vi "exprand1Lars.vi"() -> ()   [LabVIEW 2010]
uses:
  <vilib>/Analysis/NI_AALBase.lvlib
panel:
  out "Waveform Graph of random numbers":dbl[](graph)
  in  "Histogram intervals":i32
  out "Histogram":T1(graph)
  in  "Desired Expected Random Number":dbl
  in  "Number of Random Numbers":i32
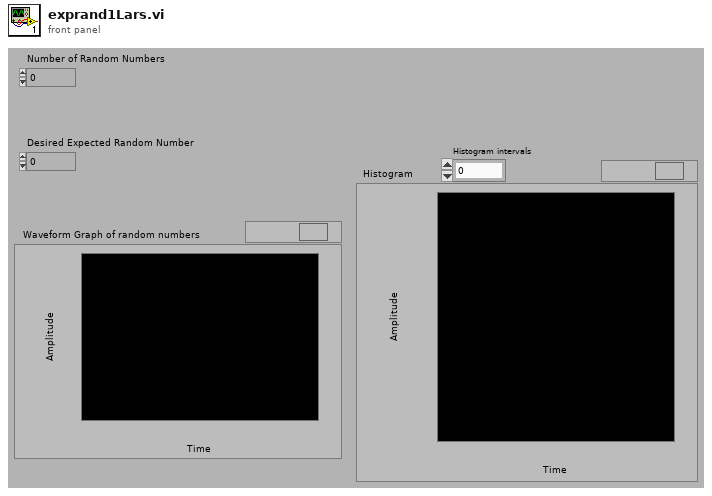
[diagram p1: front panel]
types:
  T1 = cluster{"X Values":dbl[], "Histogram: h(x)":i32[]}
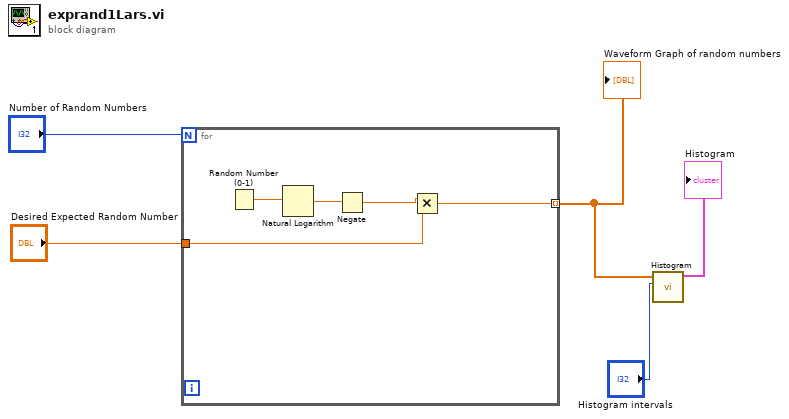
[diagram p0: block diagram]
diagram:
  n1 = for {
    N: "Number of Random Numbers" -> [_]
    tunnel: "Desired Expected Random Number" -> [w8]
    tunnel: [w7] -> w3 mode=indexing
    n2 = Random Number (0-1)() -> (number: 0 to 1=w10:dbl)
    n3 = Natural Logarithm(1:w10) -> (0:w9:dbl)
    n4 = Negate(x=w9) -> (-x=w6:dbl)
    n5 = Multiply(x=w6, y=w8) -> (x*y=w7:dbl)
  }
  "Waveform Graph of random numbers" <- w3
  n6 = call <vilib>:"Histogram.vi"("intervals"="Histogram intervals", "X"=w3) -> ("Histogram Graph"=→"Histogram":T1)  [unwired: 6 in, 3 out]
